vi "InitialiseProbeplan.vi"(8 "error in (no error)":errorcluster, 11 "ProbeStationControl in":refnum<class "ProbeStationControl.lvclass">) -> (0 "error out":errorcluster, 3 "ProbeStationControl out":refnum<class "ProbeStationControl.lvclass">)   [LabVIEW 2019]
doc: "General utility to initialise, generate, test and execute probe plans."
uses:
  InstrControl/ProbeStationControl/ProbeStationControl.lvclass
  ProbePlanParams.vi
  general_VIs/globals/QC_MeasurementSetup.vi
panel:
  in  "Continue":bool
  out "Single Needle":bool
  in  "Probe Card Channels":i32=32
  in  "Strip No.":u16(ring) items=["Strip 0", "Strip 1", "Strip 2", "Strip 3", "Strip 4", "Strip 5", "Strip 6", "Strip 7", "Strip 8", "Strip 9", "Strip 10", "Strip 11", "Strip 12", "Strip 13", "Strip 14", "Strip 15", "Strip 16", "Strip 17", "Strip 18", "Strip 19", "Strip 20", "Strip 21", "Strip 22", "Strip 23", "Strip 24", "Strip 25", "Strip 26", "Strip 27", "Strip 28", "Strip 29", "Strip 30", "Strip 31", "Strip 32", "Strip 33", "Strip 34", "Strip 35", "Strip 36", "Strip 37", "Strip 38", "Strip 39", "Strip 40", "Strip 41", "Strip 42", "Strip 43", "Strip 44", "Strip 45", "Strip 46", "Strip 47", "Strip 48", "Strip 49", "Strip 50", "Strip 51", "Strip 52", "Strip 53", "Strip 54", "Strip 55", "Strip 56", "Strip 57", "Strip 58", "Strip 59", "Strip 60", "Strip 61", "Strip 62", "Strip 63", "Strip 64", "Strip 65", "Strip 66", "Strip 67", "Strip 68", "Strip 69", "Strip 70", "Strip 71", "Strip 72", "Strip 73", "Strip 74", "Strip 75", "Strip 76", "Strip 77", "Strip 78", "Strip 79", "Strip 80", "Strip 81", "Strip 82", "Strip 83", "Strip 84", "Strip 85", "Strip 86", "Strip 87", "Strip 88", "Strip 89", "Strip 90", "Strip 91", "Strip 92", "Strip 93", "Strip 94", "Strip 95", "Strip 96", "Strip 97", "Strip 98", "Strip 99", "Strip 100", "Strip 101", "Strip 102", "Strip 103", "Strip 104", "Strip 105", "Strip 106", "Strip 107", "Strip 108", "Strip 109", "Strip 110", "Strip 111", "Strip 112", "Strip 113", "Strip 114", "Strip 115", "Strip 116", "Strip 117", "Strip 118", "Strip 119", "Strip 120", "Strip 121", "Strip 122", "Strip 123", "Strip 124", "Strip 125", "Strip 126", "Strip 127", "Strip 128", "Strip 129", "Strip 130", "Strip 131", "Strip 132", "Strip 133", "Strip 134", "Strip 135", "Strip 136", "Strip 137", "Strip 138", "Strip 139", "Strip 140", "Strip 141", "Strip 142", "Strip 143", "Strip 144", "Strip 145", "Strip 146", "Strip 147", "Strip 148", "Strip 149", "Strip 150", "Strip 151", "Strip 152", "Strip 153", "Strip 154", "Strip 155", "Strip 156", "Strip 157", "Strip 158", "Strip 159", "Strip 160", "Strip 161", "Strip 162", "Strip 163", "Strip 164", "Strip 165", "Strip 166", "Strip 167", "Strip 168", "Strip 169", "Strip 170", "Strip 171", "Strip 172", "Strip 173", "Strip 174", "Strip 175", "Strip 176", "Strip 177", "Strip 178", "Strip 179", "Strip 180", "Strip 181", "Strip 182", "Strip 183", "Strip 184", "Strip 185", "Strip 186", "Strip 187", "Strip 188", "Strip 189", "Strip 190", "Strip 191", "Strip 192", "Strip 193", "Strip 194", "Strip 195", "Strip 196", "Strip 197", "Strip 198", "Strip 199", "Strip 200", "Strip 201", "Strip 202", "Strip 203", "Strip 204", "Strip 205", "Strip 206", "Strip 207", "Strip 208", "Strip 209", "Strip 210", "Strip 211", "Strip 212", "Strip 213", "Strip 214", "Strip 215", "Strip 216", "Strip 217", "Strip 218", "Strip 219", "Strip 220", "Strip 221", "Strip 222", "Strip 223", "Strip 224", "Strip 225", "Strip 226", "Strip 227", "Strip 228", "Strip 229", "Strip 230", "Strip 231", "Strip 232", "Strip 233", "Strip 234", "Strip 235", "Strip 236", "Strip 237", "Strip 238", "Strip 239", "Strip 240", "Strip 241", "Strip 242", "Strip 243", "Strip 244", "Strip 245", "Strip 246", "Strip 247", "Strip 248", "Strip 249", "Strip 250", "Strip 251", "Strip 252", "Strip 253", "Strip 254", "Strip 255", "Strip 256", "Strip 257", "Strip 258", "Strip 259", "Strip 260", "Strip 261", "Strip 262", "Strip 263", "Strip 264", "Strip 265", "Strip 266", "Strip 267", "Strip 268", "Strip 269", "Strip 270", "Strip 271", "Strip 272", "Strip 273", "Strip 274", "Strip 275", "Strip 276", "Strip 277", "Strip 278", "Strip 279", "Strip 280", "Strip 281", "Strip 282", "Strip 283", "Strip 284", "Strip 285", "Strip 286", "Strip 287", "Strip 288", "Strip 289", "Strip 290", "Strip 291", "Strip 292", "Strip 293", "Strip 294", "Strip 295", "Strip 296", "Strip 297", "Strip 298", "Strip 299", "Strip 300", "Strip 301", "Strip 302", "Strip 303", "Strip 304", "Strip 305", "Strip 306", "Strip 307", "Strip 308", "Strip 309", "Strip 310", "Strip 311", "Strip 312", "Strip 313", "Strip 314", "Strip 315", "Strip 316", "Strip 317", "Strip 318", "Strip 319", "Strip 320", "Strip 321", "Strip 322", "Strip 323", "Strip 324", "Strip 325", "Strip 326", "Strip 327", "Strip 328", "Strip 329", "Strip 330", "Strip 331", "Strip 332", "Strip 333", "Strip 334", "Strip 335", "Strip 336", "Strip 337", "Strip 338", "Strip 339", "Strip 340", "Strip 341", "Strip 342", "Strip 343", "Strip 344", "Strip 345", "Strip 346", "Strip 347", "Strip 348", "Strip 349", "Strip 350", "Strip 351", "Strip 352", "Strip 353", "Strip 354", "Strip 355", "Strip 356", "Strip 357", "Strip 358", "Strip 359", "Strip 360", "Strip 361", "Strip 362", "Strip 363", "Strip 364", "Strip 365", "Strip 366", "Strip 367", "Strip 368", "Strip 369", "Strip 370", "Strip 371", "Strip 372", "Strip 373", "Strip 374", "Strip 375", "Strip 376", "Strip 377", "Strip 378", "Strip 379", "Strip 380", "Strip 381", "Strip 382", "Strip 383", "Strip 384", "Strip 385", "Strip 386", "Strip 387", "Strip 388", "Strip 389", "Strip 390", "Strip 391", "Strip 392", "Strip 393", "Strip 394", "Strip 395", "Strip 396", "Strip 397", "Strip 398", "Strip 399", "Strip 400", "Strip 401", "Strip 402", "Strip 403", "Strip 404", "Strip 405", "Strip 406", "Strip 407", "Strip 408", "Strip 409", "Strip 410", "Strip 411", "Strip 412", "Strip 413", "Strip 414", "Strip 415", "Strip 416", "Strip 417", "Strip 418", "Strip 419", "Strip 420", "Strip 421", "Strip 422", "Strip 423", "Strip 424", "Strip 425", "Strip 426", "Strip 427", "Strip 428", "Strip 429", "Strip 430", "Strip 431", "Strip 432", "Strip 433", "Strip 434", "Strip 435", "Strip 436", "Strip 437", "Strip 438", "Strip 439", "Strip 440", "Strip 441", "Strip 442", "Strip 443", "Strip 444", "Strip 445", "Strip 446", "Strip 447", "Strip 448", "Strip 449", "Strip 450", "Strip 451", "Strip 452", "Strip 453", "Strip 454", "Strip 455", "Strip 456", "Strip 457", "Strip 458", "Strip 459", "Strip 460", "Strip 461", "Strip 462", "Strip 463", "Strip 464", "Strip 465", "Strip 466", "Strip 467", "Strip 468", "Strip 469", "Strip 470", "Strip 471", "Strip 472", "Strip 473", "Strip 474", "Strip 475", "Strip 476", "Strip 477", "Strip 478", "Strip 479", "Strip 480", "Strip 481", "Strip 482", "Strip 483", "Strip 484", "Strip 485", "Strip 486", "Strip 487", "Strip 488", "Strip 489", "Strip 490", "Strip 491", "Strip 492", "Strip 493", "Strip 494", "Strip 495", "Strip 496", "Strip 497", "Strip 498", "Strip 499", "Strip 500", "Strip 501", "Strip 502", "Strip 503", "Strip 504", "Strip 505", "Strip 506", "Strip 507", "Strip 508", "Strip 509", "Strip 510", "Strip 511", "Strip 512", "Strip 513", "Strip 514", "Strip 515", "Strip 516", "Strip 517", "Strip 518", "Strip 519", "Strip 520", "Strip 521", "Strip 522", "Strip 523", "Strip 524", "Strip 525", "Strip 526", "Strip 527", "Strip 528", "Strip 529", "Strip 530", "Strip 531", "Strip 532", "Strip 533", "Strip 534", "Strip 535", "Strip 536", "Strip 537", "Strip 538", "Strip 539", "Strip 540", "Strip 541", "Strip 542", "Strip 543", "Strip 544", "Strip 545", "Strip 546", "Strip 547", "Strip 548", "Strip 549", "Strip 550", "Strip 551", "Strip 552", "Strip 553", "Strip 554", "Strip 555", "Strip 556", "Strip 557", "Strip 558", "Strip 559", "Strip 560", "Strip 561", "Strip 562", "Strip 563", "Strip 564", "Strip 565", "Strip 566", "Strip 567", "Strip 568", "Strip 569", "Strip 570", "Strip 571", "Strip 572", "Strip 573", "Strip 574", "Strip 575", "Strip 576", "Strip 577", "Strip 578", "Strip 579", "Strip 580", "Strip 581", "Strip 582", "Strip 583", "Strip 584", "Strip 585", "Strip 586", "Strip 587", "Strip 588", "Strip 589", "Strip 590", "Strip 591", "Strip 592", "Strip 593", "Strip 594", "Strip 595", "Strip 596", "Strip 597", "Strip 598", "Strip 599", "Strip 600", "Strip 601", "Strip 602", "Strip 603", "Strip 604", "Strip 605", "Strip 606", "Strip 607", "Strip 608", "Strip 609", "Strip 610", "Strip 611", "Strip 612", "Strip 613", "Strip 614", "Strip 615", "Strip 616", "Strip 617", "Strip 618", "Strip 619", "Strip 620", "Strip 621", "Strip 622", "Strip 623", "Strip 624", "Strip 625", "Strip 626", "Strip 627", "Strip 628", "Strip 629", "Strip 630", "Strip 631", "Strip 632", "Strip 633", "Strip 634", "Strip 635", "Strip 636", "Strip 637", "Strip 638", "Strip 639", "Strip 640", "Strip 641", "Strip 642", "Strip 643", "Strip 644", "Strip 645", "Strip 646", "Strip 647", "Strip 648", "Strip 649", "Strip 650", "Strip 651", "Strip 652", "Strip 653", "Strip 654", "Strip 655", "Strip 656", "Strip 657", "Strip 658", "Strip 659", "Strip 660", "Strip 661", "Strip 662", "Strip 663", "Strip 664", "Strip 665", "Strip 666", "Strip 667", "Strip 668", "Strip 669", "Strip 670", "Strip 671", "Strip 672", "Strip 673", "Strip 674", "Strip 675", "Strip 676", "Strip 677", "Strip 678", "Strip 679", "Strip 680", "Strip 681", "Strip 682", "Strip 683", "Strip 684", "Strip 685", "Strip 686", "Strip 687", "Strip 688", "Strip 689", "Strip 690", "Strip 691", "Strip 692", "Strip 693", "Strip 694", "Strip 695", "Strip 696", "Strip 697", "Strip 698", "Strip 699", "Strip 700", "Strip 701", "Strip 702", "Strip 703", "Strip 704", "Strip 705", "Strip 706", "Strip 707", "Strip 708", "Strip 709", "Strip 710", "Strip 711", "Strip 712", "Strip 713", "Strip 714", "Strip 715", "Strip 716", "Strip 717", "Strip 718", "Strip 719", "Strip 720", "Strip 721", "Strip 722", "Strip 723", "Strip 724", "Strip 725", "Strip 726", "Strip 727", "Strip 728", "Strip 729", "Strip 730", "Strip 731", "Strip 732", "Strip 733", "Strip 734", "Strip 735", "Strip 736", "Strip 737", "Strip 738", "Strip 739", "Strip 740", "Strip 741", "Strip 742", "Strip 743", "Strip 744", "Strip 745", "Strip 746", "Strip 747", "Strip 748", "Strip 749", "Strip 750", "Strip 751", "Strip 752", "Strip 753", "Strip 754", "Strip 755", "Strip 756", "Strip 757", "Strip 758", "Strip 759", "Strip 760", "Strip 761", "Strip 762", "Strip 763", "Strip 764", "Strip 765", "Strip 766", "Strip 767", "Strip 768", "Strip 769", "Strip 770", "Strip 771", "Strip 772", "Strip 773", "Strip 774", "Strip 775", "Strip 776", "Strip 777", "Strip 778", "Strip 779", "Strip 780", "Strip 781", "Strip 782", "Strip 783", "Strip 784", "Strip 785", "Strip 786", "Strip 787", "Strip 788", "Strip 789", "Strip 790", "Strip 791", "Strip 792", "Strip 793", "Strip 794", "Strip 795", "Strip 796", "Strip 797", "Strip 798", "Strip 799", "Strip 800", "Strip 801", "Strip 802", "Strip 803", "Strip 804", "Strip 805", "Strip 806", "Strip 807", "Strip 808", "Strip 809", "Strip 810", "Strip 811", "Strip 812", "Strip 813", "Strip 814", "Strip 815", "Strip 816", "Strip 817", "Strip 818", "Strip 819", "Strip 820", "Strip 821", "Strip 822", "Strip 823", "Strip 824", "Strip 825", "Strip 826", "Strip 827", "Strip 828", "Strip 829", "Strip 830", "Strip 831", "Strip 832", "Strip 833", "Strip 834", "Strip 835", "Strip 836", "Strip 837", "Strip 838", "Strip 839", "Strip 840", "Strip 841", "Strip 842", "Strip 843", "Strip 844", "Strip 845", "Strip 846", "Strip 847", "Strip 848", "Strip 849", "Strip 850", "Strip 851", "Strip 852", "Strip 853", "Strip 854", "Strip 855", "Strip 856", "Strip 857", "Strip 858", "Strip 859", "Strip 860", "Strip 861", "Strip 862", "Strip 863", "Strip 864", "Strip 865", "Strip 866", "Strip 867", "Strip 868", "Strip 869", "Strip 870", "Strip 871", "Strip 872", "Strip 873", "Strip 874", "Strip 875", "Strip 876", "Strip 877", "Strip 878", "Strip 879", "Strip 880", "Strip 881", "Strip 882", "Strip 883", "Strip 884", "Strip 885", "Strip 886", "Strip 887", "Strip 888", "Strip 889", "Strip 890", "Strip 891", "Strip 892", "Strip 893", "Strip 894", "Strip 895", "Strip 896", "Strip 897", "Strip 898", "Strip 899", "Strip 900", "Strip 901", "Strip 902", "Strip 903", "Strip 904", "Strip 905", "Strip 906", "Strip 907", "Strip 908", "Strip 909", "Strip 910", "Strip 911", "Strip 912", "Strip 913", "Strip 914", "Strip 915", "Strip 916", "Strip 917", "Strip 918", "Strip 919", "Strip 920", "Strip 921", "Strip 922", "Strip 923", "Strip 924", "Strip 925", "Strip 926", "Strip 927", "Strip 928", "Strip 929", "Strip 930", "Strip 931", "Strip 932", "Strip 933", "Strip 934", "Strip 935", "Strip 936", "Strip 937", "Strip 938", "Strip 939", "Strip 940", "Strip 941", "Strip 942", "Strip 943", "Strip 944", "Strip 945", "Strip 946", "Strip 947", "Strip 948", "Strip 949", "Strip 950", "Strip 951", "Strip 952", "Strip 953", "Strip 954", "Strip 955", "Strip 956", "Strip 957", "Strip 958", "Strip 959", "Strip 960", "Strip 961", "Strip 962", "Strip 963", "Strip 964", "Strip 965", "Strip 966", "Strip 967", "Strip 968", "Strip 969", "Strip 970", "Strip 971", "Strip 972", "Strip 973", "Strip 974", "Strip 975", "Strip 976", "Strip 977", "Strip 978", "Strip 979", "Strip 980", "Strip 981", "Strip 982", "Strip 983", "Strip 984", "Strip 985", "Strip 986", "Strip 987", "Strip 988", "Strip 989", "Strip 990", "Strip 991", "Strip 992", "Strip 993", "Strip 994", "Strip 995", "Strip 996", "Strip 997", "Strip 998", "Strip 999", "Strip 1000", "Strip 1001", "Strip 1002", "Strip 1003", "Strip 1004", "Strip 1005", "Strip 1006", "Strip 1007", "Strip 1008", "Strip 1009", "Strip 1010", "Strip 1011", "Strip 1012", "Strip 1013", "Strip 1014", "Strip 1015", "Strip 1016", "Strip 1017", "Strip 1018", "Strip 1019", "Strip 1020", "Strip 1021", "Strip 1022", "Strip 1023", "Strip 1024", "Strip 1025", "Strip 1026", "Strip 1027", "Strip 1028", "Strip 1029", "Strip 1030", "Strip 1031", "Strip 1032", "Strip 1033", "Strip 1034", "Strip 1035", "Strip 1036", "Strip 1037", "Strip 1038", "Strip 1039", "Strip 1040", "Strip 1041", "Strip 1042", "Strip 1043", "Strip 1044", "Strip 1045", "Strip 1046", "Strip 1047", "Strip 1048", "Strip 1049", "Strip 1050", "Strip 1051", "Strip 1052", "Strip 1053", "Strip 1054", "Strip 1055", "Strip 1056", "Strip 1057", "Strip 1058", "Strip 1059", "Strip 1060", "Strip 1061", "Strip 1062", "Strip 1063", "Strip 1064", "Strip 1065", "Strip 1066", "Strip 1067", "Strip 1068", "Strip 1069", "Strip 1070", "Strip 1071", "Strip 1072", "Strip 1073", "Strip 1074", "Strip 1075", "Strip 1076", "Strip 1077", "Strip 1078", "Strip 1079", "Strip 1080", "Strip 1081", "Strip 1082", "Strip 1083", "Strip 1084", "Strip 1085", "Strip 1086", "Strip 1087", "Strip 1088", "Strip 1089", "Strip 1090", "Strip 1091", "Strip 1092", "Strip 1093", "Strip 1094", "Strip 1095", "Strip 1096", "Strip 1097", "Strip 1098", "Strip 1099", "Strip 1100", "Strip 1101", "Strip 1102", "Strip 1103", "Strip 1104", "Strip 1105", "Strip 1106", "Strip 1107", "Strip 1108", "Strip 1109", "Strip 1110", "Strip 1111", "Strip 1112", "Strip 1113", "Strip 1114", "Strip 1115", "Strip 1116", "Strip 1117", "Strip 1118", "Strip 1119", "Strip 1120", "Strip 1121", "Strip 1122", "Strip 1123", "Strip 1124", "Strip 1125", "Strip 1126", "Strip 1127", "Strip 1128", "Strip 1129", "Strip 1130", "Strip 1131", "Strip 1132", "Strip 1133", "Strip 1134", "Strip 1135", "Strip 1136", "Strip 1137", "Strip 1138", "Strip 1139", "Strip 1140", "Strip 1141", "Strip 1142", "Strip 1143", "Strip 1144", "Strip 1145", "Strip 1146", "Strip 1147", "Strip 1148", "Strip 1149", "Strip 1150", "Strip 1151", "Strip 1152", "Strip 1153"]
  out "Probeplan:":string
  in  "Region":u16(ring) items=["Segment_1", "Segment_2"]
  in  "New Button":bool
  in  "Jump Button":bool
  # "Probeplan"
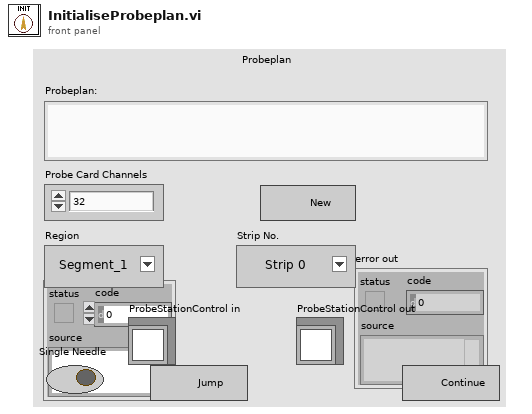
[diagram p1: front panel]
types:
  T1 = enum8{"Enabled", "Disabled", "Disabled and Grayed Out"}
  T2 = cluster{"Strip Number OUT":i32, "X0":i32, "Y0":i32, "X1":i32, "Y1":i32, "Xref":dbl, "Yref":dbl, "ProbePlan type":u32, "Inner pads offset":ext, "Outer pads offset":ext, "l_inner":ext, "l_outer":ext, "strip numbering":u16, "Device Orientation":ext, "Stagger offset":i32, "Yoffset":dbl, "Strip pitch":dbl, "Fiducail separation":dbl, "Radius":ext, "Relative strip angles":dbl, "Probeplan description":string, "ProbePlan array":cluster{"Region":string, "ProbePoints":cluster{"X":dbl, "Y":dbl, "Label":string, "CardViable?":bool}[]}[], "Test ProbePoints":cluster{"Regions Enabled":bool[], "From index":u32[], "To index":u32[]}}
  T3 = cluster{"Bias Supply":refnum<class "SupplyControl.lvclass">, "SMU":refnum<class "SupplyControl.lvclass">, "LCR":refnum<class "LCRControl.lvclass">, "Probe Card Channels":i32, "Bias Voltage [V]":dbl, "First strip":i32, "Last strip":i32, "Base Voltage [V]":dbl, "Base Ramp Step [V]":dbl, "Base Ramp Interval [ms]":u32, "High Voltage [V]":dbl, "High Ramp Step [V]":dbl, "High Ramp Interval [ms]":u32, "AC frequency [Hz]":i32, "AC amplitude [V]":dbl, "RC Configuration":u16, "Single Needle":bool, "Temperature Readout":enum16{"Read Arduino", "Enter manually"}, "Arduino":refnum<class "ArduinoControl.lvclass">, "Fraction of good strips [%]":dbl, "ProbeStation":refnum<class "ProbeStationControl.lvclass">, "Switching":refnum<class "Switching.lvclass">, "Matrix used?":bool, "Matrix X Channels":cluster{"Bias Supply / SMU LO":i32, "Bias Supply / SMU HI":i32, "CV Box LO":i32, "CV Box HI":i32, "CV Box LO IN":i32, "CV Box HI IN":i32, "Volt meter LO":i32, "Volt meter HI":i32, "Mux1 C1":i32, "Mux1 C2":i32, "Mux2 C1":i32, "Mux2 C2":i32}, "Pinholes Y/N":bool, "Capacitance Y/N":bool, "Resistance Y/N":bool, "Bias Supply Name":string, "SMU Name":string, "LCR Name":string}
  T4 = cluster{"Region":string, "ProbePoints":cluster{"X":dbl, "Y":dbl, "Label":string, "CardViable?":bool}[]}[]
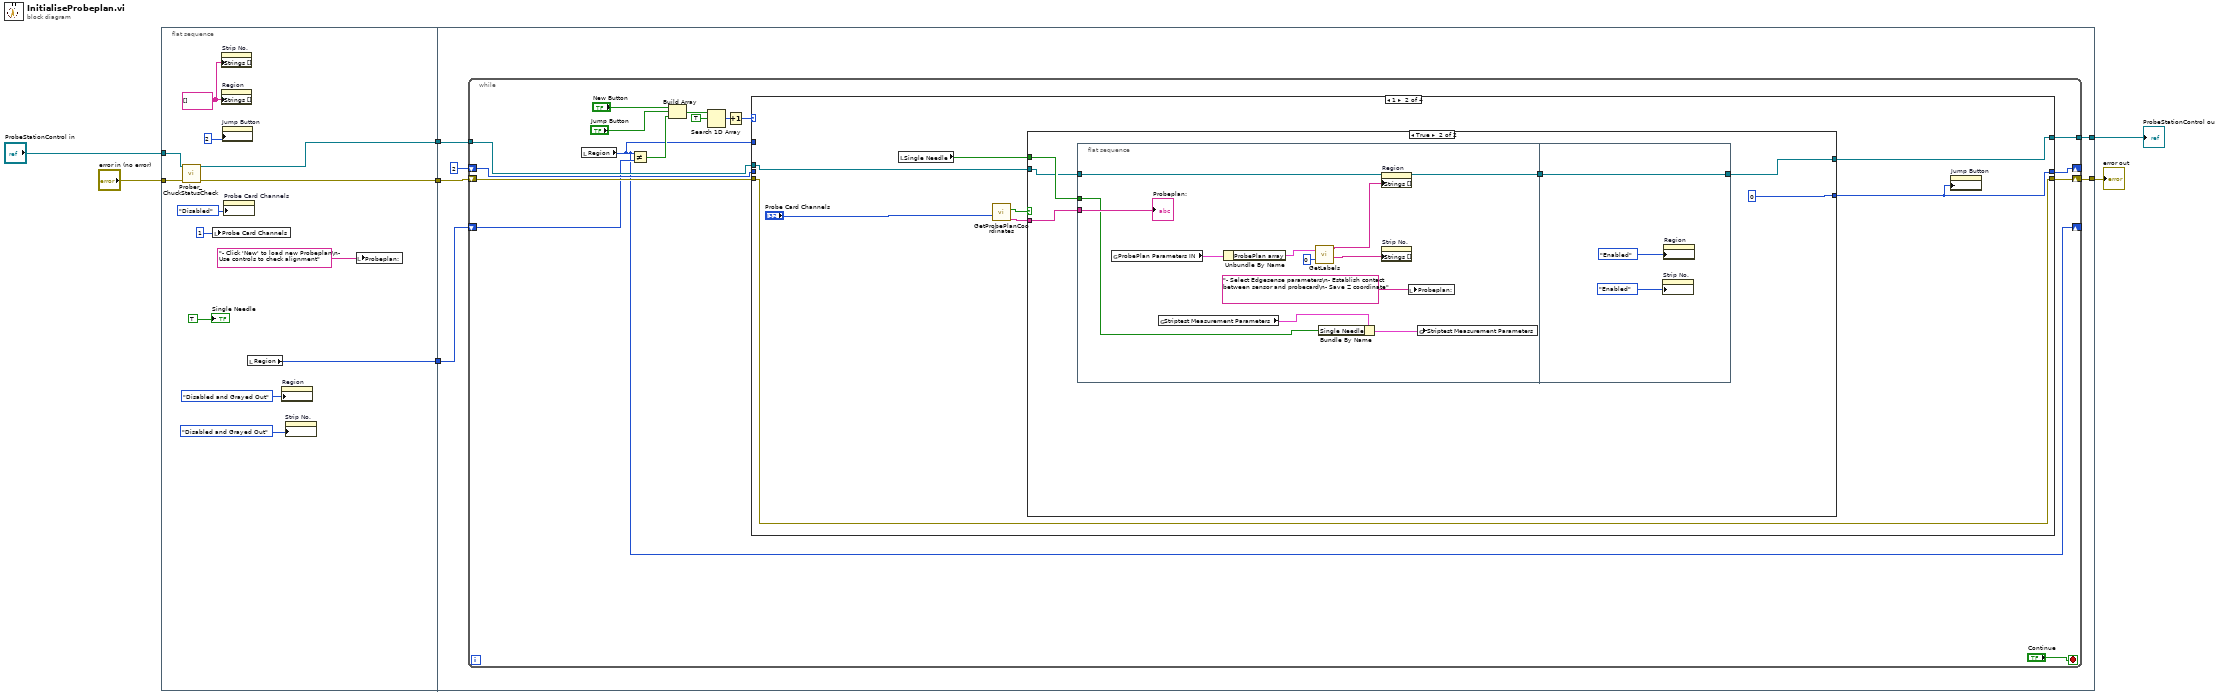
[diagram p0: block diagram]
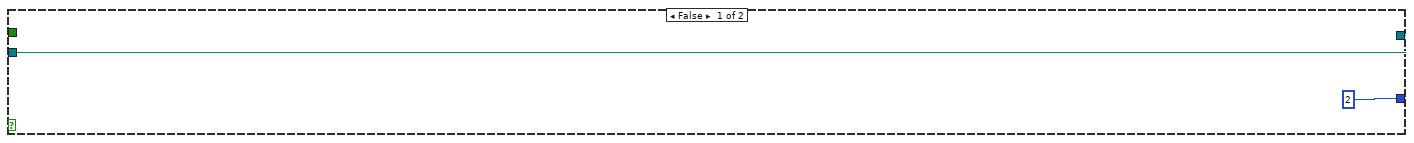
[diagram p3: hidden frame]
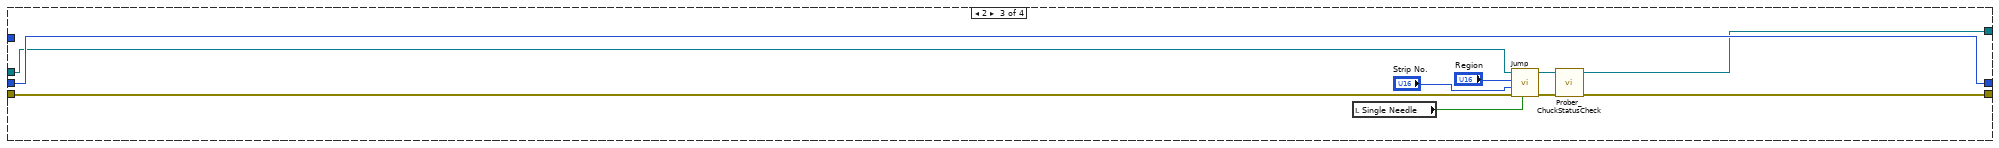
[diagram p4: hidden frame]
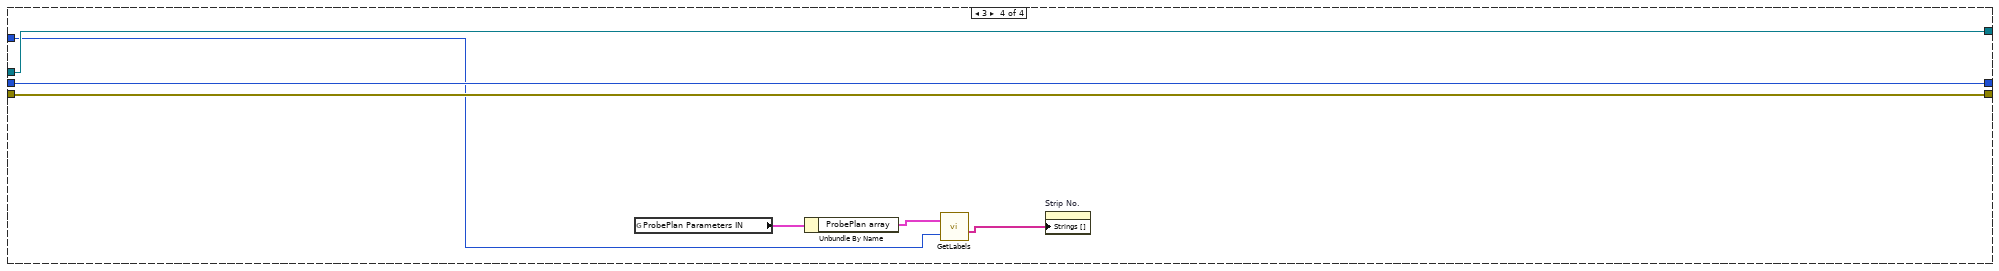
[diagram p5: hidden frame]
diagram:
  n1 = flat-sequence {
    tunnel: "ProbeStationControl in" -> [w17]
    tunnel: [w14] -> w4
    tunnel: "error in (no error)" -> [w16]
    tunnel: [w15] -> w3
    tunnel: [w8] -> w1
    tunnel: w4 -> [w25]
    tunnel: [w24] -> w6
    tunnel: w3 -> [w23]
    tunnel: [w22] -> w2
    tunnel: w1 -> [w21]
    frame #0 {
      w18 = string[] []
      n2 = call-dynamic "Prober_ChuckStatusCheck.vi"("error in (no error)"=w16, "ProbeStationControl in"=w17) -> ("error out"=w15:errorcluster, "ProbeStationControl out"=w14:refnum<class "ProbeStationControl.lvclass">)  [unwired: 7 in, 1 out]
      n3 = local write "Probe Card Channels"(1 ("Probe Card Channels")) -> ()
      n4 = property on="Strip No." class="Ring (strict)"("Strings []"=w18) -> ()  [unwired: 2 in, 2 out]
      n5 = property on="Region" class="Ring (strict)"("Strings []"=w18) -> ()  [unwired: 2 in, 2 out]
      n6 = property on="Jump Button" class="Bool"("DisabledEnum"=2) -> ()  [unwired: 2 in, 2 out]
      n7 = property on="Probe Card Channels" class="DigNum (strict)"("DisabledEnum"=T1."Disabled" ("Disabled")) -> ()  [unwired: 2 in, 2 out]
      n8 = local read "Region"() -> (w8:u16)
      n9 = property on="Region" class="Ring (strict)"("DisabledEnum"=T1."Disabled and Grayed Out" ("Disabled")) -> ()  [unwired: 2 in, 2 out]
      n10 = property on="Strip No." class="Ring (strict)"("DisabledEnum"=T1."Disabled and Grayed Out" ("Disabled")) -> ()  [unwired: 2 in, 2 out]
      n11 = local write "Probeplan:"("- Click 'New' to load new Probeplan\n- Use controls to check alignment") -> ()
      "Single Needle" <- TRUE ("Single Needle")
    }
    frame #1 {
      n12 = while {
        shift-right: [w37] -> _
        shift-left: 2 -> [w38]
        tunnel: w25 -> [w35]
        tunnel: [w34] -> w24
        shift-right: [w32] -> w22
        shift-left: w23 -> [w33]
        shift-right: [w27] -> _
        shift-left: w21 -> [w29]
        stop <- "Continue" stop-if-true
        n13 = local read "Region"() -> (w27:u16)
        n14 = Not Equal?(x=w27, y=w29) -> (x != y?=w28:bool)
        n15 = Build Array("New Button", "Jump Button", w28) -> (w41:bool[])
        n16 = Search 1D Array(1D array=w41, element=TRUE) -> (index of element=w42:i32)  [unwired: 1 in]
        n17 = Increment(x=w42) -> (x+1=w39:i32)
        n18 = case shown="1" w39 {
          tunnel: w38 -> [w45 _ w85 w89]
          tunnel: [w45 w53 w85 w89] -> w37
          tunnel: w35 -> [w44 w51 w84 w91]
          tunnel: [w44 w50 w83 w91] -> w34
          tunnel: w33 -> [w43 w49 w79 w90]
          tunnel: [w43 w49 w81 w90] -> w32
          tunnel: w27 -> [_ _ _ w86]
          frame 0, Default {
          }
          frame 1 {
            n19 = local read "Single Needle"() -> (w48:bool)
            n20 = call "GetProbePlanCoordinates.vi"("Probe Card Channels"="Probe Card Channels") -> ("file path"=w46:string, "OK?"=w47:bool)  [unwired: 1 out]
            n21 = case shown="True" w47 {
              tunnel: [2 0] -> w53
              tunnel: w46 -> [_ w59]
              tunnel: w51 -> [w54 w57]
              tunnel: [w54 w60] -> w50
              tunnel: w48 -> [_ w58]
              frame False {
              }
              frame True {
                n22 = flat-sequence {
                  tunnel: w59 -> [w68]
                  tunnel: w58 -> [w67]
                  tunnel: w57 -> [w66]
                  tunnel: [w66] -> w56
                  tunnel: [w75] -> w60
                  tunnel: w56 -> [w75]
                  frame #0 {
                    n23 = global read "ProbePlanParams.vi" "ProbePlan Parameters IN"() -> (w70:T2)
                    n24 = global read "QC_MeasurementSetup.vi" "Striptest Measurement Parameters"() -> (w71:T3)
                    n25 = Unbundle By Name(w70) -> ("ProbePlan array"=w65:T4)
                    n26 = call "GetLabels.vi"("Array"=w65, "Region of Interest"=0) -> ("Region Labels"=w63:string[], "Strip Labels"=w62:string[])  [unwired: 2 out]
                    n27 = Bundle By Name(cluster=w71, "Single Needle"=w67) -> (w72:T3)
                    n28 = property on="Region" class="Ring (strict)"("Strings []"=w63) -> ()  [unwired: 2 in, 2 out]
                    n29 = property on="Strip No." class="Ring (strict)"("Strings []"=w62) -> ()  [unwired: 2 in, 2 out]
                    n30 = local write "Probeplan:"("- Select Edgesense parameters\n- Establish contact between sensor and probecard\n- Save Z coordinate") -> ()
                    n31 = global write "QC_MeasurementSetup.vi" "Striptest Measurement Parameters"(w72) -> ()
                    "Probeplan:" <- w68
                  }
                  frame #1 {
                    n32 = property on="Strip No." class="Ring (strict)"("DisabledEnum"=T1."Enabled" ("Disabled")) -> ()  [unwired: 2 in, 2 out]
                    n33 = property on="Region" class="Ring (strict)"("DisabledEnum"=T1."Enabled" ("Disabled")) -> ()  [unwired: 2 in, 2 out]
                  }
                }
              }
            }
            n34 = property on="Jump Button" class="Bool"("DisabledEnum"=w53) -> ()  [unwired: 2 in, 2 out]
          }
          frame 2 {
            n35 = local read "Single Needle"() -> (w76:bool)
            n36 = call "Jump.vi"("Single Needle"=w76, "Error In"=w79, "Strip No."="Strip No.", "Region"="Region", "ProbeStationControl in"=w84) -> ("Error Out"=w80:errorcluster, "ProbeStationControl out"=w82:refnum<class "ProbeStationControl.lvclass">)  [unwired: 5 in]
            n37 = call-dynamic "Prober_ChuckStatusCheck.vi"("error in (no error)"=w80, "ProbeStationControl in"=w82) -> ("error out"=w81:errorcluster, "ProbeStationControl out"=w83:refnum<class "ProbeStationControl.lvclass">)  [unwired: 7 in, 1 out]
          }
          frame 3 {
            n38 = global read "ProbePlanParams.vi" "ProbePlan Parameters IN"() -> (w92:T2)
            n39 = Unbundle By Name(w92) -> ("ProbePlan array"=w87:T4)
            n40 = call "GetLabels.vi"("Array"=w87, "Region of Interest"=w86) -> ("Strip Labels"=w88:string[])  [unwired: 3 out]
            n41 = property on="Strip No." class="Ring (strict)"("Strings []"=w88) -> ()  [unwired: 2 in, 2 out]
          }
        }
      }
    }
  }
  "ProbeStationControl out" <- w6
  "error out" <- w2
